vi "00_MOD_Control_Loops.vi"(8 "error in":errorcluster, 11 "Main Config File Refnum":T3) -> (0 "error out":errorcluster)   [LabVIEW 2018]
doc: "Control Loops Module for NGTS.\nThis Vi runs the Control Expressions for the PID Loops and other custom control requiring hardcoded LabVIEW G code to perform. Expression evaluations occur in the Tag Manager Module.\n\n2007_11 Mike Ashe\nmichael.ashe@imaginatics.net\nCell: 860-961-0876"
uses:
  <vilib>/Utility/config.llb/Config Data RefNum.ctl
  <vilib>/Platform/TimedLoop/XDataNode/timing_clust.ctl
  <vilib>/Platform/TimedLoop/XDataNode/nitl_modes.ctl
  <vilib>/Platform/TimedLoop/XDataNode/wakeup.ctl
  Common/Controls/NGTS_PID Loop Tag and Gain Set.ctl
  <vilib>/Utility/config.llb/Read Key (String).vi
  <vilib>/Platform/TimedLoop/XDataNode/XDataNode.xnode
  <vilib>/Utility/config.llb/NI_LVConfig.lvlib
  <vilib>/Platform/TimedLoop/XDataNode/XDNodeRunTimeDep.lvlib
panel:
  out "In Range?":bool=TRUE
  in  "Tab Control":T1(tab)=enum."Module Status & Errors"
  in  "Wait On Error?":bool
  in  "Error Wait(mS)":i32=1000
  out "Current Error":i32
  out "Error Array":errorcluster[](array[cluster]) caption="Status        Error Code                   Error Source"
  in  "Error Action":T2(radio)
  out "# Errors":i32
  # "NGTS Icon"
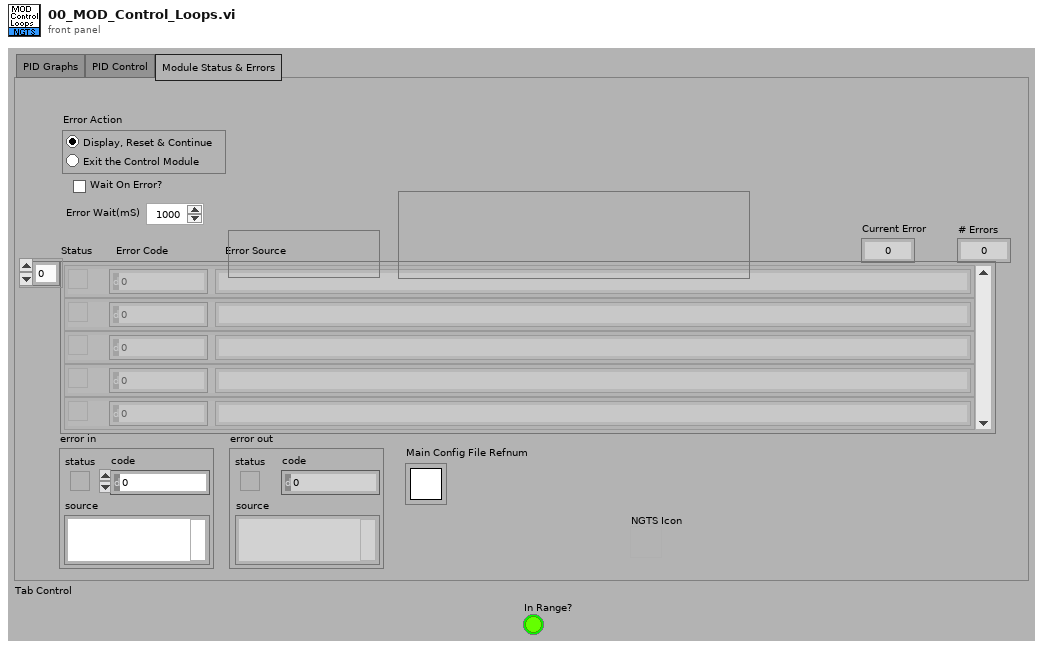
[diagram p1: front panel]
types:
  T1 = enum32{"PID Graphs", "PID Control", "Module Status & Errors"}
  T2 = enum32{"Display, Reset & Continue", "Exit the Control Module"}
  T3 = typedef "NI_LVConfig.lvlib/Config Data RefNum.ctl" = refnum<k1>
  T4 = typedef "Control_Loops Shift Variables.ctl" = cluster{"error":errorcluster, "queue data":T5, "WDT Time Stamp 1":timestamp, "Q_TO":i32, "LogErrors?":bool, "Tag Set Directory":path, "LogPath":path, "PID Tag Sets":T6[], "PIDChartRef":refnum<vi>, "Loop SP-PVs":cluster{"Loop N":cluster{dbl, dbl}, "Picture":picture}[], "WDT_TO":i32}
  T5 = typedef "Command Queue Cluster.ctl" = cluster{"Command":string, "Variant Data":variant}
  T6 = typedef "NGTS_PID Loop Tag and Gain Set.ctl" = cluster{"PID Loop#":i32, "PID Vars Tags":string[], "PID GS Tags":string[], "Loop Name":string}
  T7 = typedef "XDNodeRunTimeDep.lvlib/timing_clust.ctl" = cluster{"Expected End [f-1]":u64, "Actual End [f-1]":u64, "Finished Late? [f-1]":bool, "Expected End [i-1]":u64, "Actual End [i-1]":u64, "Finished Late? [i-1]":bool, "Expected Start [i]":u64, "Actual Start [i]":u64, "Expected Start [f]":u64, "Actual Start [f]":u64, "Source Name":string, "Structure Name":string, "Period":i64, "Deadline":i64, "Offset":i64, "Start":i64, "Priority":i32, "Timeout":i32, "Mode":T8, "Wakeup Reason":T9, "Error":errorcluster, "Source Type":string, "Secondary Source Type":string, "Global End Time":u64, "Global Start Time":u64, "Frame Duration":u64, "Iteration Duration":u64, "Assigned CPU":i32, "I/O Scan Engine Mode":u32}
  T8 = typedef "XDNodeRunTimeDep.lvlib/nitl_modes.ctl" = enum32{"No Change", "Process missed periods, maintain original phase", "Discard missed periods, maintain original phase", "Process missed periods, ignore original phase", "Discard missed periods, ignore original phase"}
  T9 = typedef "XDNodeRunTimeDep.lvlib/wakeup.ctl" = enum32{"Normal", "Aborted", "Asynchronous wakeup", "Timing source error", "Timed loop error", "Timeout"}
  T10 = enum16{"get data", "set all data", "set Process Variable", "initialize"}
  T11 = enum16{"get data", "set manual data", "set automatic data", "Set Mode", "initialize"}
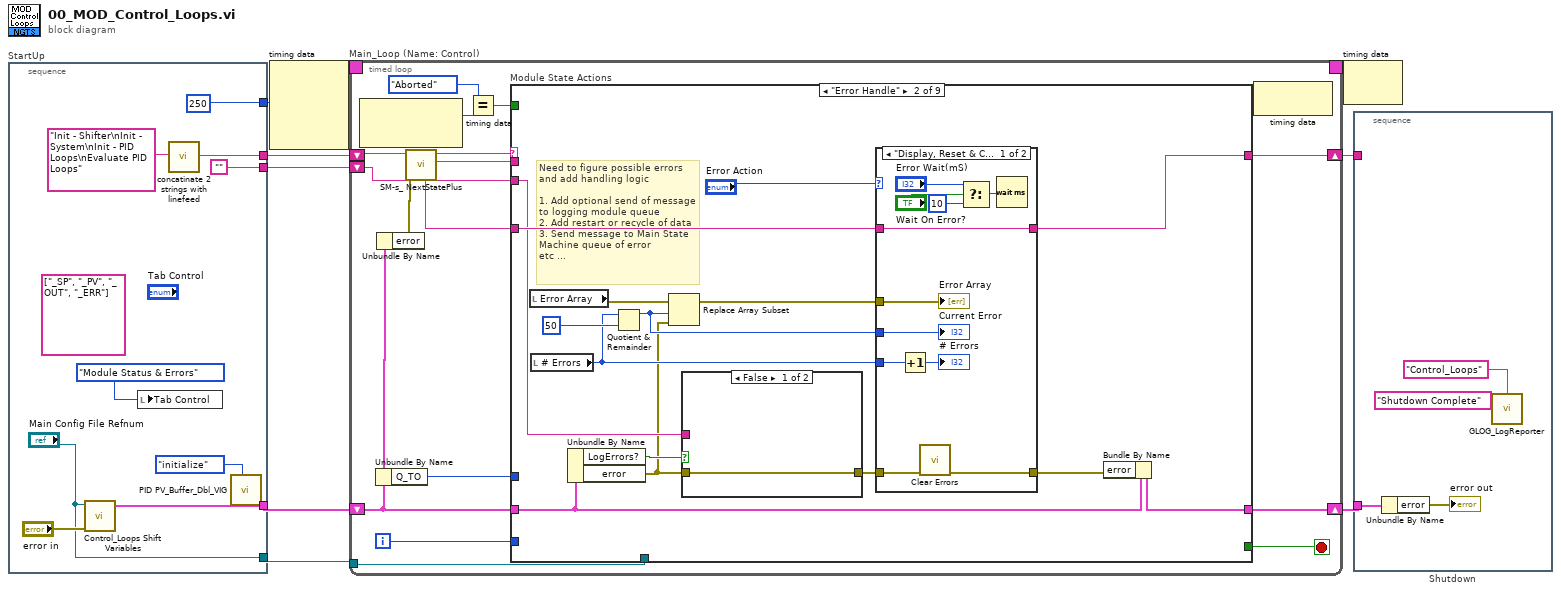
[diagram p0: block diagram]
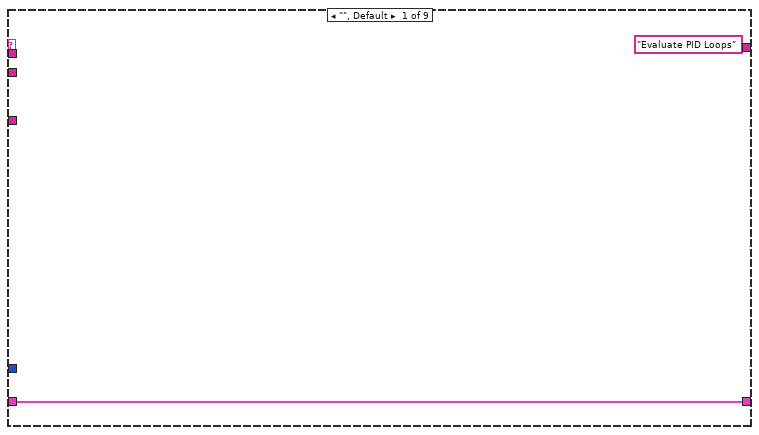
[diagram p2: hidden frame]
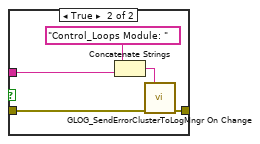
[diagram p3: hidden frame]
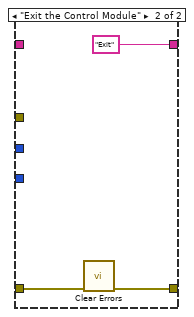
[diagram p4: hidden frame]
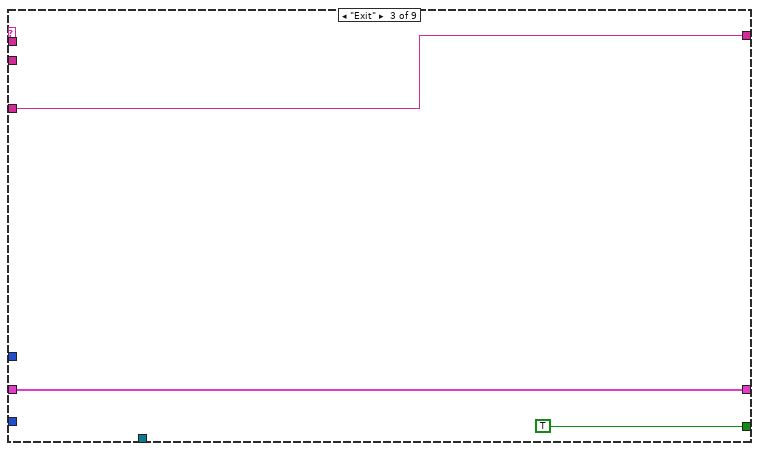
[diagram p5: hidden frame]
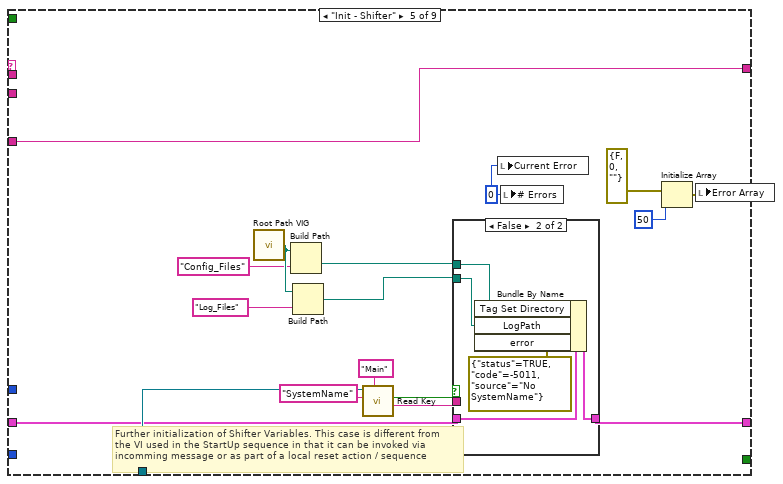
[diagram p7: hidden frame]
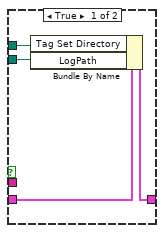
[diagram p8: hidden frame]
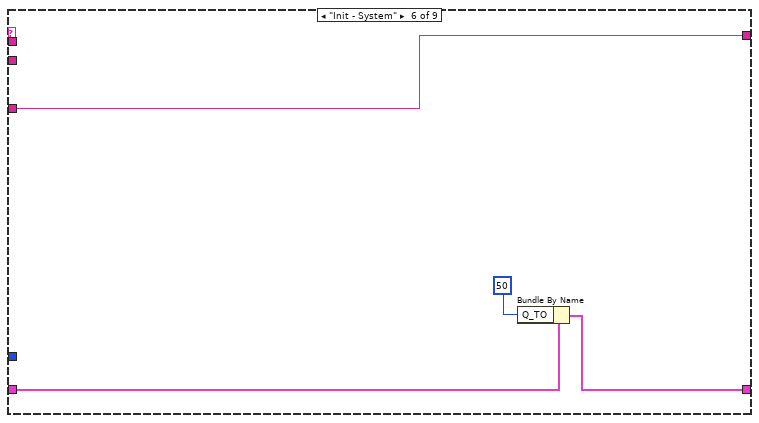
[diagram p9: hidden frame]
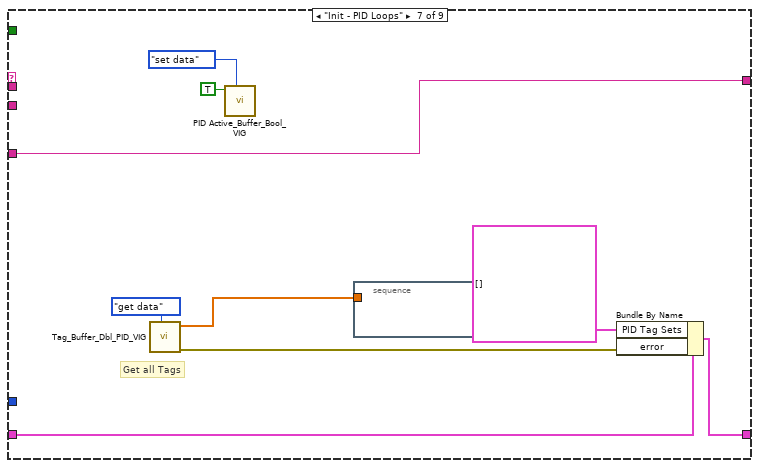
[diagram p10: hidden frame]
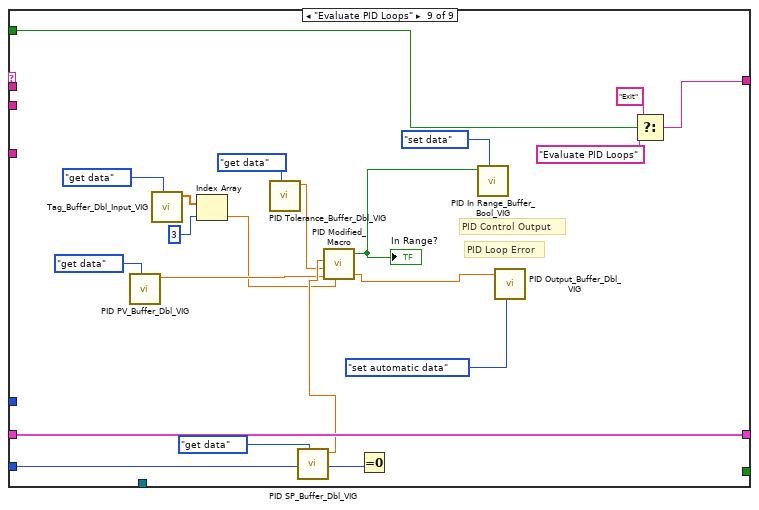
[diagram p12: hidden frame]
diagram:
  n1 = stacked-sequence "StartUp" {
    tunnel: [w15] -> w9
    tunnel: [w16] -> w7
    tunnel: ["Main Config File Refnum"] -> w5
    tunnel: [""] -> w4
    tunnel: [u32 250 ("milliseconds to wait")] -> w1
    frame #0 {
      (unwired) string[] ["_SP", "_PV", "_OUT", "_ERR"]
      n2 = call "Control_Loops Shift Variables.vi"("error in"="error in", "Main Config File Refnum"="Main Config File Refnum") -> ("VARS Control_Loops"=w15:T4)  [unwired: 8 in, 1 out]
      n3 = local write "Tab Control"(T1."Module Status & Errors" ("Tab Control")) -> ()
      n4 = call "concatinate 2 strings with linefeed.vi"("String 1"="Init - Shifter\nInit - System\nInit - PID Loops\nEvaluate PID Loops") -> ("Concatinated OUT"=w16:string)  [unwired: 7 in]
      n5 = call "PID PV_Buffer_Dbl_VIG.vi"("Operation"=enum16{"get data", "set data", "initialize"}."initialize") -> ()  [unwired: 9 in, 2 out]
    }
  }
  n6 = node-c288(w1) -> (w3:T7)  [unwired: 3 in]
  n7 = timed-loop "Main_Loop (Name: Control)" {
    shift-right: [w33] -> w8
    shift-left: w9 -> [w31]
    shift-right: [w29] -> w6
    shift-left: w7 -> [w27]
    tunnel: w5 -> [w23]
    shift-left: w4 -> [w22]
    timing: w3 -> [_]
    timing-out: [_] -> w2
    i -> [w34]
    stop <- w32 stop-if-true
    n8 = node-c288() -> (w20:T9)  [unwired: 1 in, 1 out]
    n9 = Unbundle By Name(w31) -> ("Q_TO"=w30:i32)
    n10 = Unbundle By Name(w31) -> ("error"=w28:errorcluster)
    n11 = call "SM-s_ NextStatePlus.vi"("error?"=w28, "States String"=w27) -> ("Argument"=w25:string, "Current State"=w26:string, "Next States"=w24:string)  [unwired: 7 in]
    n12 = Equal?(x=wakeup."Aborted" ("Wakeup Reason"), y=w20) -> (x = y?=w19:bool)
    n13 = case "Module State Actions" shown="\"Error Handle\"" w26 {
      tunnel: w25 -> [_ _ _ _ _ _ _ _ _]
      tunnel: w34 -> [_ _ _ _ _ _ _ _ w132]
      tunnel: w31 -> [w38 w53 w76 w79 w81 w108 w117 w119 w140]
      tunnel: [w38 w52 w76 w79 w90 w107 w116 w119 w140] -> w33
      tunnel: [_ _ TRUE _ _ _ _ _ _] -> w32
      tunnel: w24 -> [_ w50 w75 w78 w96 w109 w118 w120 _]
      tunnel: w30 -> [_ _ _ _ _ _ _ _ _]
      tunnel: ["Evaluate PID Loops" w49 w75 w78 w96 w109 w118 w120 w138] -> w29
      tunnel: w23 -> [_ _ _ _ w91 _ _ _ _]
      tunnel: w22 -> [_ w41 _ _ _ _ _ _ _]
      tunnel: w19 -> [_ _ _ _ _ _ _ _ w136]
      frame "", Default {
      }
      frame "Error Handle" {
        # "Need to figure possible errors and add handling logic\n\n1. Add optional send of message to logging module queue\n2. Add restart or recycle of data\n3. Send message to Main State Machine queue of error\netc ..."
        n14 = local read "Error Array"() -> (w48:errorcluster[])
        n15 = local read "# Errors"() -> (w45:i32)
        n16 = Unbundle By Name(w53) -> ("LogErrors?"=w42:bool, "error"=w40:errorcluster)
        n17 = Quotient & Remainder(x=w45, y=50 ("dimension size")) -> (x-y*floor(x/y)=w44:i32)  [unwired: 1 out]
        n18 = Replace Array Subset(array=w48, new element=w40, index=w44) -> (w47:errorcluster[])
        n19 = case shown="False" w42 {
          tunnel: w40 -> [w55 w60]
          tunnel: [w55 w59] -> w43
          tunnel: w41 -> [_ w56]
          frame False {
          }
          frame True {
            n20 = Concatenate Strings("Control_Loops Module: " ("System"), w56) -> (w58:string)
            n21 = call "GLOG_SendErrorClusterToLogMngr On Change.vi"("System"=w58, "error in"=w60) -> ("error out"=w59:errorcluster)  [unwired: 13 in]
          }
        }
        n22 = case shown="\"Display, Reset & Continue\", Default" "Error Action" {
          tunnel: [w71 w72] -> w54
          tunnel: w43 -> [w70 w73]
          tunnel: w50 -> [w69 _]
          tunnel: [w69 "Exit" ("Next States")] -> w49
          tunnel: w47 -> [w68 _]
          tunnel: w45 -> [w67 _]
          tunnel: w44 -> [w65 _]
          frame "Display, Reset & Continue", Default {
            n23 = Increment(x=w67) -> (x+1=→"# Errors":i32)
            n24 = call <vilib>:"Clear Errors.vi"("error in (no error)"=w70) -> ("error out"=w71:errorcluster)  [unwired: 5 in, 1 out]
            n25 = Select(t="Error Wait(mS)", s="Wait On Error?", f=10) -> (s? t:f=w64:i32)
            n26 = Wait (ms)(milliseconds to wait=w64) -> ()  [unwired: 1 out]
            "Current Error" <- w65
            "Error Array" <- w68
          }
          frame "Exit the Control Module" {
            n27 = call <vilib>:"Clear Errors.vi"("error in (no error)"=w73) -> ("error out"=w72:errorcluster)  [unwired: 5 in, 1 out]
          }
        }
        n28 = Bundle By Name(cluster=w53, "error"=w54) -> (w52:T4)
      }
      frame "Exit" {
      }
      frame "----- Initialization Actions -----" {
        # "This frame should never actually run. It is used to delineate the\ngroupings in the State machine"
      }
      frame "Init - Shifter" {
        w89 = 0 ("# Errors")
        # "Further initialization of Shifter Variables. This case is different from\nthe VI used in the StartUp sequence in that it can be invoked via\nincomming message or as part of a local reset action / sequence"
        n29 = call "Root Path VIG.vi"() -> ("Root VI's Path"=w85:path)  [unwired: 1 in]
        n30 = Build Path(base path=w85, name or relative path="Config_Files") -> (appended path=w80:path)
        n31 = Build Path(base path=w85, name or relative path="Log_Files") -> (appended path=w82:path)
        n32 = call-poly <vilib>:"Read Key.vi"("section"="Main", "key"="SystemName", "refnum"=w91) -> ("value"=w94:string, "found?"=w95:bool)  [unwired: 5 in, 2 out]
        n33 = case shown="False" w95 {
          tunnel: [w100 w105] -> w90
          tunnel: w80 -> [w99 w104]
          tunnel: w81 -> [w98 w103]
          tunnel: w82 -> [w97 w102]
          tunnel: w94 -> [_ _]
          frame True {
            n34 = Bundle By Name(cluster=w98, "Tag Set Directory"=w99, "LogPath"=w97) -> (w100:T4)
          }
          frame False {
            n35 = Bundle By Name(cluster=w103, "Tag Set Directory"=w104, "LogPath"=w102, "error"=errorcluster {"status"=TRUE, "code"=-5011, "source"="No SystemName"} ("error out")) -> (w105:T4)
          }
        }
        n36 = local write "Current Error"(w89) -> ()
        n37 = local write "# Errors"(w89) -> ()
        n38 = Initialize Array(errorcluster {"status"=FALSE, "code"=0, "source"=""} ("error out"), 50 ("dimension size")) -> (w88:errorcluster[])
        n39 = local write "Error Array"(w88) -> ()
      }
      frame "Init - System" {
        n40 = Bundle By Name(cluster=w108, "Q_TO"=50) -> (w107:T4)
      }
      frame "Init - PID Loops" {
        # "Get all Tags"
        n41 = call "Tag_Buffer_Dbl_PID_VIG.vi"("Operation"=T10."get data") -> ("error out"=w115:errorcluster, "tag_data_out"=w113:dbl[])  [unwired: 9 in]
        n42 = call "PID Active_Buffer_Bool_VIG.vi"("Operation"=enum16{"get data", "set data", "initialize"}."set data", "Boolean"=TRUE) -> ()  [unwired: 8 in, 2 out]
        n43 = stacked-sequence {
          tunnel: w113 -> [_]
          frame #0 {
          }
        }
        n44 = Bundle By Name(cluster=w117, "PID Tag Sets"=T6[] [], "error"=w115) -> (w116:T4)
      }
      frame "----- Control Actions -----" {
        # "This frame should never actually run. It is used to delineate the\ngroupings in the State machine"
      }
      frame "Evaluate PID Loops" {
        # "PID Loop Error"
        # "PID Control Output"
        n45 = call "PID PV_Buffer_Dbl_VIG.vi"("Operation"=enum16{"get data", "set data", "initialize"}."get data") -> ("Numeric"=w130:dbl)  [unwired: 9 in, 1 out]
        n46 = call "Tag_Buffer_Dbl_Input_VIG.vi"("Operation"=enum16{"get data", "set data", "initialize"}."get data") -> ("tag_data_out"=w125:dbl[])  [unwired: 9 in, 1 out]
        n47 = Index Array(array=w125, index=3) -> (element=w122:dbl)
        n48 = call "PID Tolerance_Buffer_Dbl_VIG.vi"("Operation"=enum16{"get data", "set data", "initialize"}."get data") -> ("Numeric"=w127:dbl)  [unwired: 9 in, 1 out]
        n49 = call "PID SP_Buffer_Dbl_VIG.vi"("Operation"=enum16{"get data", "set data", "initialize"}."get data") -> ("Numeric"=w131:dbl)  [unwired: 9 in, 1 out]
        n50 = call "PID Modified_Macro.vi"("Diff Press Setpoint"=w131, "Supply Pressure"=w122, "Tolerance"=w127, "Differential Pressure"=w130) -> ("In Range?"=w129:bool, "BP Output"=w121:dbl)  [unwired: 5 in]
        "In Range?" <- w129
        n51 = Equal To 0?(x=w132) -> ()  [unwired: 1 out]
        n52 = call "PID In Range_Buffer_Bool_VIG.vi"("Operation"=enum16{"get data", "set data", "initialize"}."set data", "Boolean"=w129) -> ()  [unwired: 7 in, 3 out]
        n53 = call "PID Output_Buffer_Dbl_VIG.vi"("Operation"=T11."set automatic data", "Numeric"=w121) -> ()  [unwired: 8 in, 2 out]
        n54 = Select(t="Exit", s=w136, f="Evaluate PID Loops") -> (s? t:f=w138:string)
      }
    }
    n55 = node-c288() -> ()  [unwired: 1 in, 1 out]
  }
  n56 = node-c288(w2) -> ()  [unwired: 1 out]
  n57 = stacked-sequence "Shutdown" {
    tunnel: w8 -> [w144]
    tunnel: w6 -> [_]
    frame #0 {
      n58 = Unbundle By Name(w144) -> ("error"=→"error out":errorcluster)
      n59 = call "GLOG_LogReporter.vi"("Log Entry"="Shutdown Complete", "System Name"="Control_Loops" ("Module Name")) -> ()  [unwired: 12 in, 2 out]
    }
  }
